vi "ACQ Device create channels.vi"(7 "Config analog chanells new":T1, 11 "device in":tag) -> (2 "DAQ analog Array":tag[](array[tag]), 3 "DAQ digital Array":tag[](array[tag]))   [LabVIEW 2013]
uses:
  Kontrolki/KartaDAQ/ACQ analog channel config.ctl
  Kontrolki/KartaDAQ/ACQ analog channel config new.ctl
panel:
  out "DAQ cont":tag
  out "DAQ digital":tag
  out "DAQ analog":tag
  in  "Config analog chanells":T2
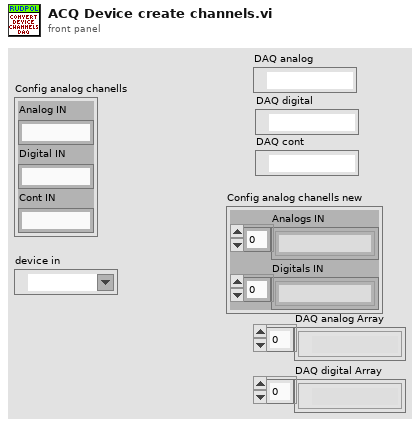
[diagram p1: front panel]
types:
  T1 = typedef "ACQ analog channel config new.ctl" = cluster{"Analogs IN":string[], "Digitals IN":string[]}
  T2 = typedef "ACQ analog channel config.ctl" = cluster{"Analog IN":string, "Digital IN":string, "Cont IN":string}
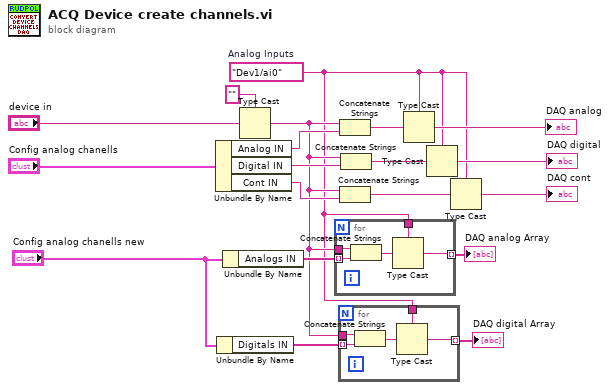
[diagram p0: block diagram]
diagram:
  w3 = tag "Dev1/ai0"  # Analog Inputs
  n1 = Unbundle By Name("Config analog chanells") -> ("Analog IN"=w15:string, "Digital IN"=w16:string, "Cont IN"=w17:string)
  n2 = Unbundle By Name("Config analog chanells new") -> ("Digitals IN"=w5:string[])
  n3 = Unbundle By Name("Config analog chanells new") -> ("Analogs IN"=w7:string[])
  n4 = Type Cast(type="", x="device in") -> (*(type *) &x=w4:string)
  n5 = for {
    tunnel: w7 -> [w24] mode=indexing
    tunnel: w4 -> [w23]
    tunnel: w3 -> [w21]
    tunnel: [w20] -> w2 mode=indexing
    n6 = Concatenate Strings(w23, w24) -> (w22:string)
    n7 = Type Cast(type=w21, x=w22) -> (*(type *) &x=w20:tag)
  }
  "DAQ analog Array" <- w2
  n8 = for {
    tunnel: w5 -> [w29] mode=indexing
    tunnel: w4 -> [w28]
    tunnel: w3 -> [w26]
    tunnel: [w25] -> w1 mode=indexing
    n9 = Concatenate Strings(w28, w29) -> (w27:string)
    n10 = Type Cast(type=w26, x=w27) -> (*(type *) &x=w25:tag)
  }
  "DAQ digital Array" <- w1
  n11 = Concatenate Strings(w4, w15) -> (w6:string)
  n12 = Concatenate Strings(w4, w17) -> (w19:string)
  n13 = Concatenate Strings(w4, w16) -> (w18:string)
  n14 = Type Cast(type=w3, x=w6) -> (*(type *) &x=→"DAQ analog":tag)
  n15 = Type Cast(type=w3, x=w18) -> (*(type *) &x=→"DAQ digital":tag)
  n16 = Type Cast(type=w3, x=w19) -> (*(type *) &x=→"DAQ cont":tag)
